vi "Register GUI.vi"(3 "error in (no error)":errorcluster) -> (0 "error out":errorcluster, 1 "REG ARRAy":u32[](array[numeric])=[6826, 65535, 65535, 65535, 32768, 320, 13312])   [LabVIEW 2012]
panel:
  in  "Register Adress 96":bool[](array[boolean])=[FALSE, TRUE, FALSE, TRUE, FALSE, TRUE, FALSE, TRUE, FALSE, TRUE, FALSE, TRUE, TRUE, FALSE, FALSE, FALSE]
  out "REG 96":u32=6826
  out "?":bool[](array[boolean])=[TRUE, TRUE, TRUE, TRUE, TRUE, TRUE, TRUE, TRUE, TRUE, TRUE, TRUE, TRUE, TRUE, TRUE, TRUE, TRUE, FALSE, FALSE, FALSE, FALSE, FALSE, FALSE, FALSE, FALSE, FALSE, FALSE, FALSE, FALSE, FALSE, FALSE, FALSE, FALSE, FALSE, FALSE, FALSE, FALSE, FALSE, FALSE, FALSE, FALSE, FALSE, FALSE, FALSE, FALSE, FALSE, FALSE, FALSE, FALSE, FALSE, FALSE, FALSE, FALSE, FALSE, FALSE, FALSE, FALSE, FALSE, FALSE, FALSE, FALSE, FALSE, FALSE, FALSE, FALSE]
  out "REG 99":u32=65535
  in  "DAC_TH1":u32=255
  in  "DAC_TH4":u32=255
  out "?":bool[](array[boolean])=[TRUE, TRUE, TRUE, TRUE, TRUE, TRUE, TRUE, TRUE, TRUE, TRUE, TRUE, TRUE, TRUE, TRUE, TRUE, TRUE, FALSE, FALSE, FALSE, FALSE, FALSE, FALSE, FALSE, FALSE, FALSE, FALSE, FALSE, FALSE, FALSE, FALSE, FALSE, FALSE, FALSE, FALSE, FALSE, FALSE, FALSE, FALSE, FALSE, FALSE, FALSE, FALSE, FALSE, FALSE, FALSE, FALSE, FALSE, FALSE, FALSE, FALSE, FALSE, FALSE, FALSE, FALSE, FALSE, FALSE, FALSE, FALSE, FALSE, FALSE, FALSE, FALSE, FALSE, FALSE]
  out "REG 98":u32=65535
  in  "DAC_TH0":u32=255
  in  "DAC_TH3":u32=255
  out "?":bool[](array[boolean])=[TRUE, TRUE, TRUE, TRUE, TRUE, TRUE, TRUE, TRUE, TRUE, TRUE, TRUE, TRUE, TRUE, TRUE, TRUE, TRUE, FALSE, FALSE, FALSE, FALSE, FALSE, FALSE, FALSE, FALSE, FALSE, FALSE, FALSE, FALSE, FALSE, FALSE, FALSE, FALSE, FALSE, FALSE, FALSE, FALSE, FALSE, FALSE, FALSE, FALSE, FALSE, FALSE, FALSE, FALSE, FALSE, FALSE, FALSE, FALSE, FALSE, FALSE, FALSE, FALSE, FALSE, FALSE, FALSE, FALSE, FALSE, FALSE, FALSE, FALSE, FALSE, FALSE, FALSE, FALSE]
  out "REG 97":u32=65535
  in  "DAC_TH2":u32=255
  in  "DAC_TH5":u32=255
  in  "Register Adress 102":bool[](array[boolean])=[FALSE, FALSE, FALSE, FALSE, FALSE, FALSE, FALSE, FALSE, FALSE, FALSE, TRUE, FALSE, TRUE, TRUE, FALSE, FALSE]
  out "REG 102":u32=13312
  in  "Register Adress 101":bool[](array[boolean])=[FALSE, FALSE, FALSE, FALSE, FALSE, FALSE, TRUE, TRUE, TRUE, TRUE, TRUE, FALSE, FALSE, FALSE, FALSE, FALSE]
  out "REG 101":u32=320
  in  "Register Adress 100":bool[](array[boolean])=[FALSE, FALSE, FALSE, FALSE, FALSE, FALSE, FALSE, FALSE, FALSE, FALSE, FALSE, FALSE, FALSE, FALSE, FALSE, TRUE]
  out "REG 100":u32=32768
  # "0           1            2"
  # "Unused"
  # "DAC_TH0"
  # "DAC_TH1"
  # "DAC_TH2"
  # "DAC_TH3"
  # "DAC_TH4"
  # "DAC_TH5"
  # "DAC_MUX_ENA"
  # "Register Adress 97"
  # "Register Adress 98"
  # "Register Adress 99"
  # "a         b         c"
  # "a         b         c"
  # "a         b         c"
  # "a         b         c"
  # "a         b         c"
  # "Unused"
  # "CH0"
  # "CH1"
  # "CH2"
  # "CH3"
  # "CH4"
  # "a         b         c"
  # "ENA_0  ENA_1"
  # "ENA_0  ENA_1"
  # "a         b         c"
  # "BUFF\nENA"
  # "R       E       S      E        R     V        E      D"
  # "MUX"
  # "LVDS"
  # "CH5"
  # "CH6"
  # "R               E               S               E                  R                V             E              D"
  # "0            1            2            3           4             5"
  # "DAC _IB"
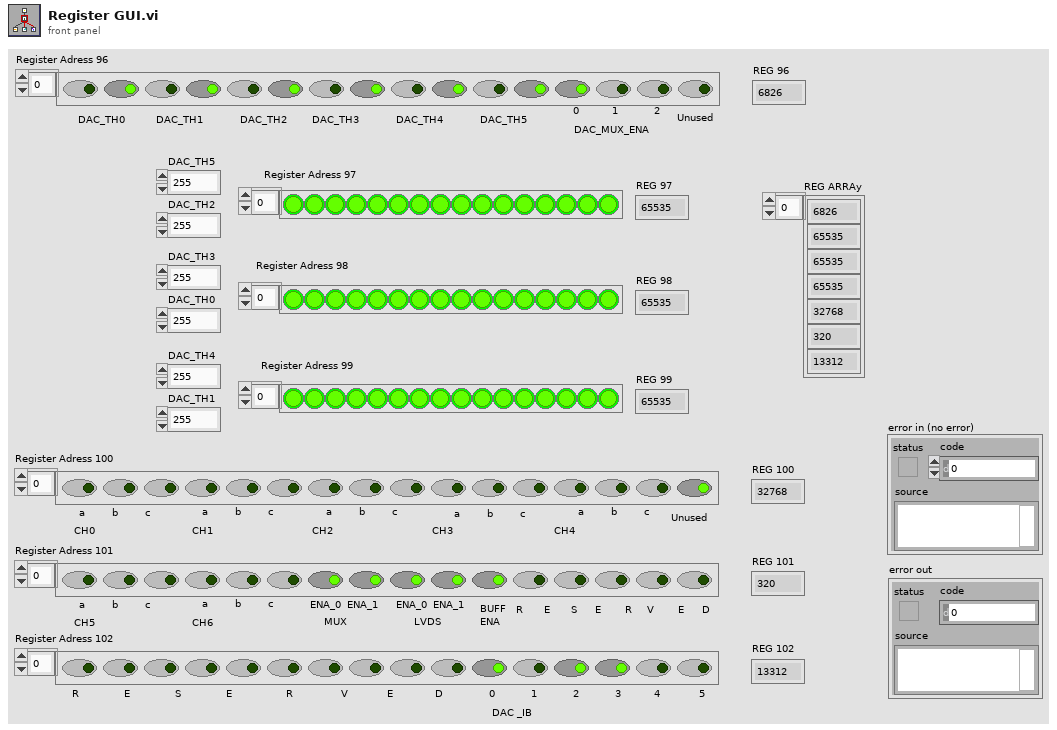
[diagram p1: front panel]
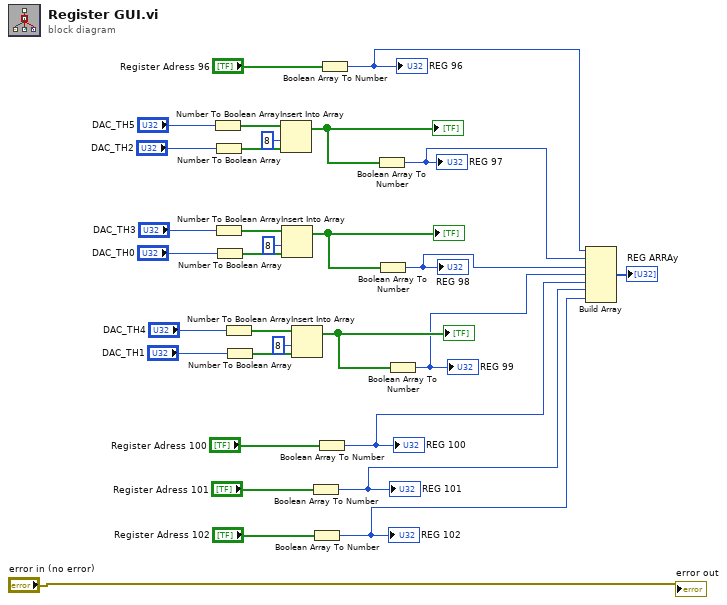
[diagram p0: block diagram]
diagram:
  n1 = Number To Boolean Array(number="DAC_TH5") -> (Boolean array=w26:bool[])
  n2 = Number To Boolean Array(number="DAC_TH2") -> (Boolean array=w25:bool[])
  n3 = Number To Boolean Array(number="DAC_TH3") -> (Boolean array=w20:bool[])
  n4 = Number To Boolean Array(number="DAC_TH0") -> (Boolean array=w19:bool[])
  n5 = Number To Boolean Array(number="DAC_TH4") -> (Boolean array=w14:bool[])
  n6 = Number To Boolean Array(number="DAC_TH1") -> (Boolean array=w13:bool[])
  n7 = Insert Into Array(array=w26, index=8, new element=w25) -> (w24:bool[])
  "?" <- w24
  n8 = Insert Into Array(array=w20, index=8, new element=w19) -> (w18:bool[])
  "?" <- w18
  n9 = Insert Into Array(array=w14, index=8, new element=w13) -> (w12:bool[])
  "?" <- w12
  n10 = Boolean Array To Number(Boolean array="Register Adress 101") -> (number=w4:u32)
  "REG 101" <- w4
  n11 = Boolean Array To Number(Boolean array="Register Adress 102") -> (number=w3:u32)
  "REG 102" <- w3
  n12 = Boolean Array To Number(Boolean array="Register Adress 100") -> (number=w5:u32)
  "REG 100" <- w5
  n13 = Boolean Array To Number(Boolean array="Register Adress 96") -> (number=w9:u32)
  "REG 96" <- w9
  n14 = Boolean Array To Number(Boolean array=w24) -> (number=w8:u32)
  "REG 97" <- w8
  n15 = Boolean Array To Number(Boolean array=w18) -> (number=w7:u32)
  "REG 98" <- w7
  n16 = Boolean Array To Number(Boolean array=w12) -> (number=w6:u32)
  "REG 99" <- w6
  n17 = Build Array(w9, w8, w7, w6, w5, w4, w3) -> (→"REG ARRAy":u32[])
  "error out" <- "error in (no error)"
